vi "Doc_parse.vi"() -> ()   [LabVIEW 2018]
uses:
  <vilib>/ATEsystem/CLAUDIE_xlsx/Excel_class/Read_excel/Open xlsx.vi
  <vilib>/LVH/i3 JSON/JSON Generation/Create Value Files/Create Value - Object.vi
  <vilib>/LVH/i3 JSON/JSON Generation/Add Object Parameter Files/Add Object Parameter - String.vi
  <vilib>/xml/Close Reference(Node).vi
  VS/labview test/x64/Release/Dll1.dll
  <vilib>/xml/NI_XML.lvlib
  <resource>/objmgr/DOMUserDefRef.rc
  <vilib>/ATEsystem/CLAUDIE_xlsx/Excel_class/Excel_class.lvclass
  <vilib>/LVH/i3 JSON/i3-json.lvlib
panel:
  in  "Name 2":string="header2"
  in  "input variable 2":i8=5
  in  "input variable":i8
  in  "b":i32=5
  in  "a":i32=1
  out "json output":string
  in  "Name":string="header1"
  out "Sheet_name":string
  out "Shared_strings":string[][](array[string])
  in  "List_index":i32
  in  "File Path":path=path "C:/LabviewFiles/LabView/Projects/1259_usbComm/specsheetsConsole/Sheets/ConsoleProcedures.xlsx"
  in  "XPath expression":string="/Config/FeatureArray/FeatureItem"
  in  "XML File Path":path=path "C:/LabviewFiles/LabView/learning(Lee)/LVU examples/xmlParsing/ETNT22116.xml"
  out "XML":string
  out "Search Results":string[](array[string])
  out "output variable":i32
  out "return":string
  out "return type":i32
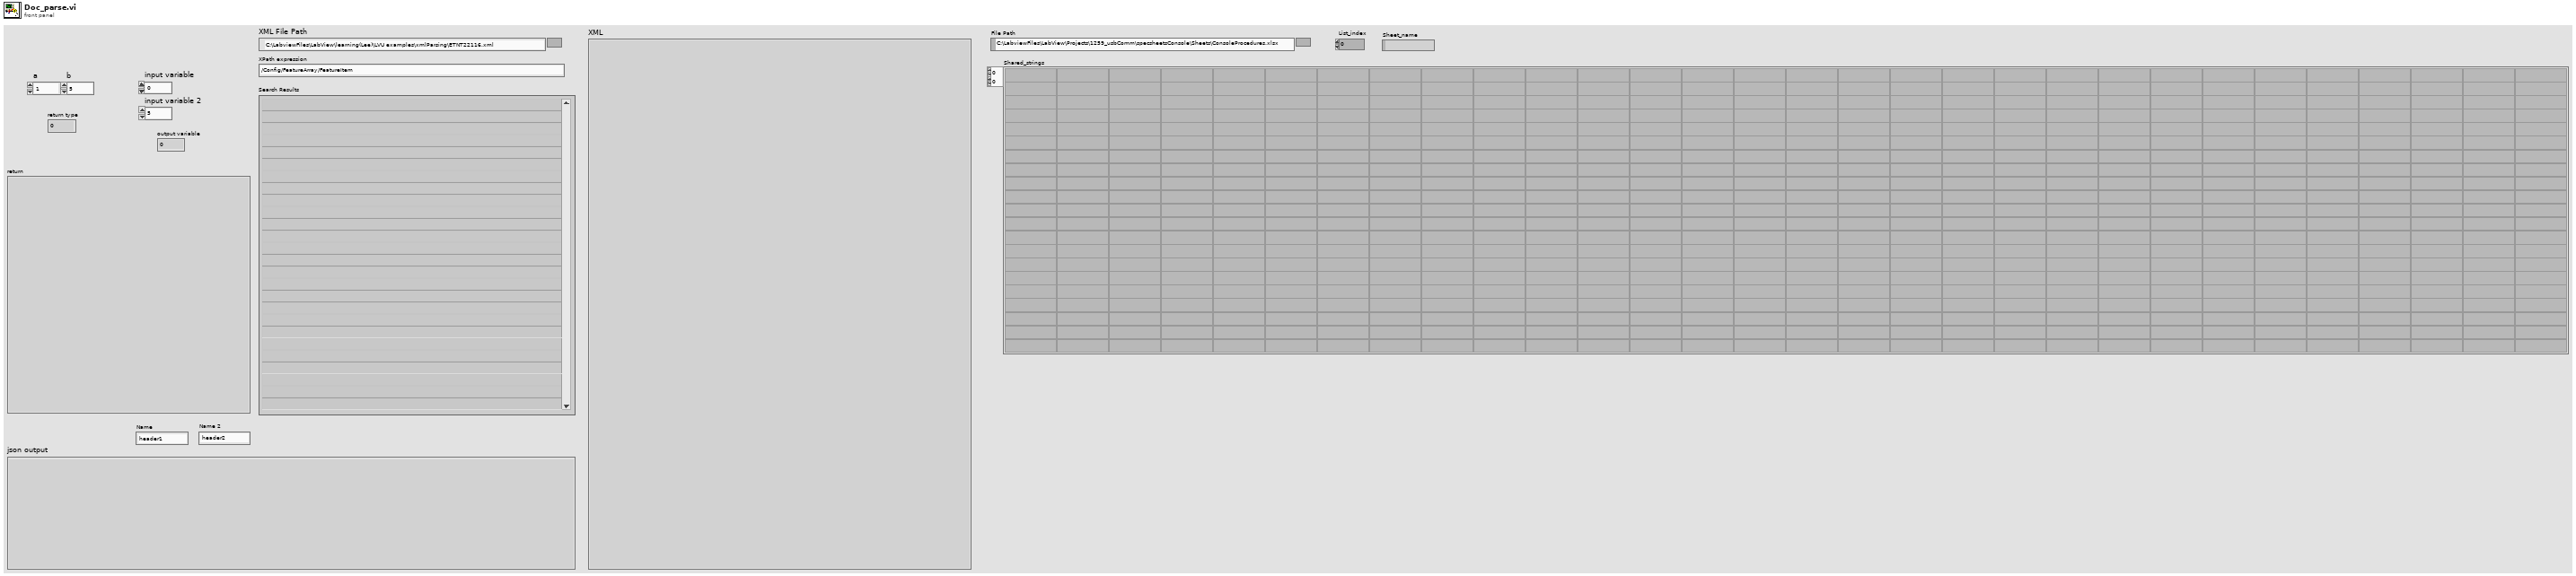
[diagram p1: front panel]
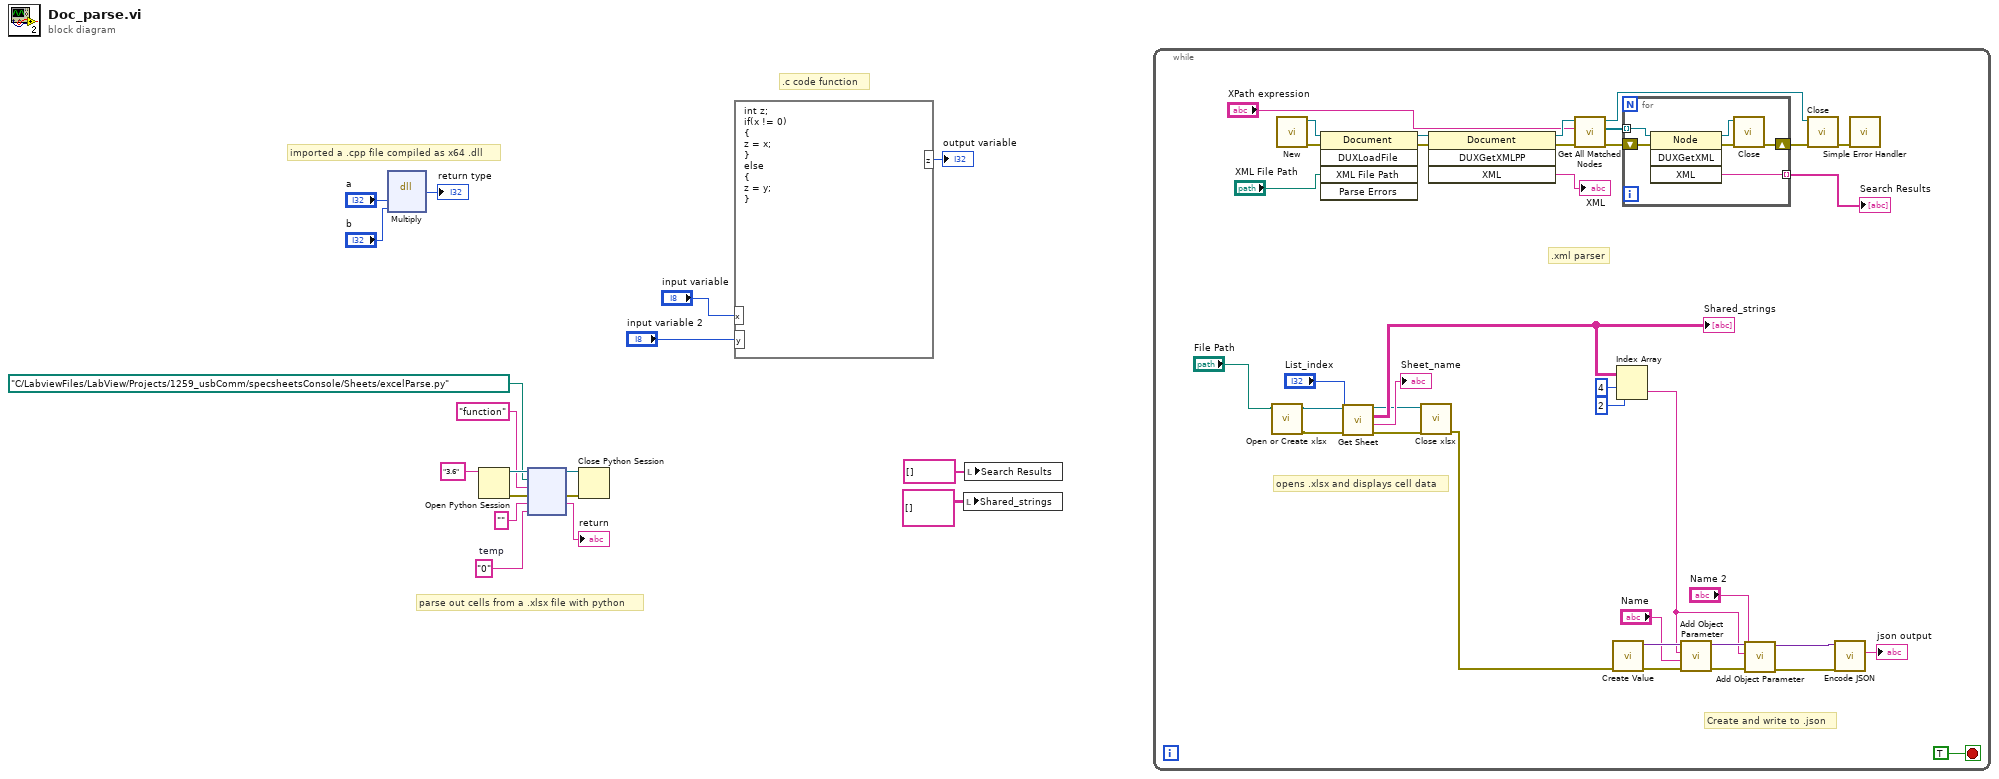
[diagram p0: block diagram]
diagram:
  w6 = "0"  # temp
  # ".c code function"
  # "parse out cells from a .xlsx file with python"
  # "imported a .cpp file compiled as x64 .dll"
  n1 = dll-call lib="C:/LabviewFiles/LabView/learning(Lee)/LVU examples/VS/labview test/x64/Release/Dll1.dll" fn="Multiply"("a"="a", "b"="b") -> ("return type"=→"return type":i32)  [unwired: 5 in, 2 out]
  n2 = Open Python Session(python version="3.6" ("Python version")) -> (session out=w15:refnum<k35>, error out=w13:errorcluster)  [unwired: 2 in]
  n3 = node(w15, path "C:/LabviewFiles/LabView/Projects/1259_usbComm/specsheetsConsole/Sheets/excelParse.py" ("module path"), "function" ("function name"), w13, "", w6) -> (w8:refnum<k35>, w7:errorcluster, →"return":string)  [unwired: 1 in, 2 out]
  n4 = Close Python Session(session in=w8, error in=w7) -> ()  [unwired: 1 out]
  n5 = formula code="int z;\nif(x != 0)\n{\nz = x;\n}\nelse\n{\nz = y;\n}"("x"="input variable", "y"="input variable 2") -> ("z"=→"output variable":i32)
  n6 = local write "Shared_strings"(string[][] [] ("Shared_strings")) -> ()
  n7 = local write "Search Results"(string[] [] ("Search Results")) -> ()
  n8 = while {
    stop <- TRUE stop-if-true
    # "Create and write to .json"
    # "opens .xlsx and displays cell data"
    # ".xml parser"
    n9 = call-poly <vilib>:"Open or Create xlsx.vi"("File Path"="File Path") -> ("error out"=w19:errorcluster, "Excel_class"=w20:refnum<class "Excel_class.lvclass">)  [unwired: 9 in]
    n10 = call <vilib>:"New.vi"() -> ("error out"=w48:errorcluster, "DOM document out"=w47:refnum<k20>)  [unwired: 8 in]
    n11 = invoke class="Document" method="DUXLoadFile"(reference=w47, error in=w48, "XML File Path"="XML File Path") -> (reference out=w50:refnum<k20>, error out=w49:errorcluster)  [unwired: 2 in, 3 out]
    n12 = call <vilib>:"Get Sheet.vi"("error in (no error)"=w19, "List_index"="List_index", "Excel_class"=w20) -> ("error out"=w23:errorcluster, "Sheet_name"=→"Sheet_name":string, "Shared_strings"=w38:string[][], "Excel_class"=w24:refnum<class "Excel_class.lvclass">)  [unwired: 5 in]
    "Shared_strings" <- w38
    n13 = call <vilib>:"Close xlsx.vi"("error in (no error)"=w23, "Excel_class"=w24) -> ("error out"=w22:errorcluster)  [unwired: 9 in]
    n14 = invoke class="Document" method="DUXGetXMLPP"(reference=w50, error in=w49) -> (reference out=w46:refnum<k20>, error out=w44:errorcluster, "XML"=→"XML":string)  [unwired: 2 in, 1 out]
    n15 = call <vilib>:"Get All Matched Nodes.vi"("error in (no error)"=w44, "XPath expression"="XPath expression", "node in"=w46) -> ("error out"=w54:errorcluster, "node result array"=w55:refnum<k20>[], "node out"=w52:refnum<k20>)  [unwired: 6 out]
    n16 = call-poly <vilib>:"Create Value.vi"("error in (no error)"=w22) -> ("error out"=w34:errorcluster, "JSON Tree"=w35:variant)  [unwired: 9 in]
    n17 = Index Array(array=w38, index (row)=4, index (col)=2 ("disabled index (col)")) -> (element=w30:string)
    n18 = for {
      tunnel: w55 -> [w57] mode=indexing
      shift-right: [w59] -> w53
      shift-left: w54 -> [w58]
      tunnel: [w56] -> w42 mode=indexing
      n19 = invoke on="Invoke Node" class="Node" method="DUXGetXML"(reference=w57, error in=w58) -> (reference out=w60:refnum<k20>, error out=w61:errorcluster, "XML"=w56:string)  [unwired: 2 in, 1 out]
      n20 = call-poly <vilib>:"Close.vi"("error in (no error)"=w61, "node"=w60) -> ("error out"=w59:errorcluster)  [unwired: 7 out]
    }
    "Search Results" <- w42
    n21 = call-poly <vilib>:"Add Object Parameter.vi"("error in (no error)"=w34, "Name"="Name", "String"=w30, "JSON Tree in (JSON Object)"=w35) -> ("error out"=w28:errorcluster, "JSON Tree out (JSON Object)"=w31:variant)  [unwired: 6 in]
    n22 = call-poly <vilib>:"Add Object Parameter.vi"("error in (no error)"=w28, "Name"="Name 2", "String"=w30, "JSON Tree in (JSON Object)"=w31) -> ("error out"=w26:errorcluster, "JSON Tree out (JSON Object)"=w27:variant)  [unwired: 6 in]
    n23 = call-poly <vilib>:"Close.vi"("error in (no error)"=w53, "node"=w52) -> ("error out"=w51:errorcluster)  [unwired: 7 out]
    n24 = call <vilib>:"Encode JSON.vi"("error in (no error)"=w26, "JSON Tree"=w27) -> ("String"=→"json output":string)  [unwired: 4 in, 1 out]
    n25 = call <vilib>:"Simple Error Handler.vi"("error in (no error)"=w51) -> ()  [unwired: 1 in, 8 out]
  }
